vi "SET_PEG_LEG.vi"(10 "argv":string[](array[string]), 11 "args":u8) -> ()   [LabVIEW 2011]
uses:
  joe_johnson/peg_leg_state.ctl
panel:
  in  "StateMaps":cluster{"Name":string, "State":T1}[](array[cluster])=[{"Name"="up", "State"=enum."up"}, {"Name"="down", "State"=enum."down"}, {"Name"="unfold", "State"=enum."unfold"}]
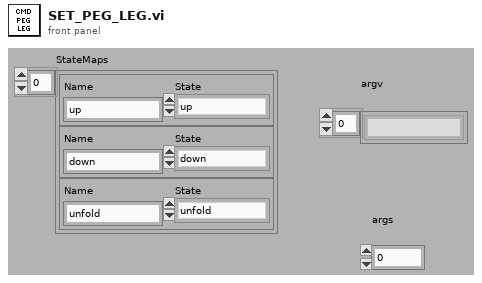
[diagram p1: front panel]
types:
  T1 = typedef "peg_leg_state.ctl" = enum16{"up", "down", "unfold", "manual"}
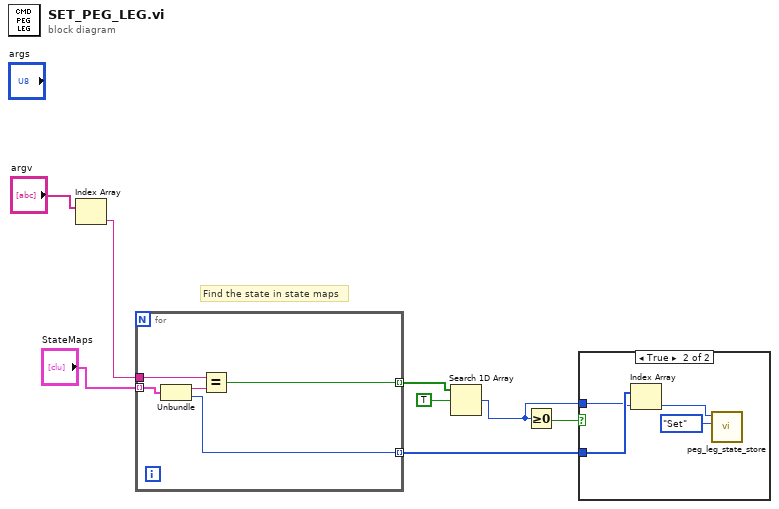
[diagram p0: block diagram]
diagram:
  # "Find the state in state maps"
  n1 = Index Array(array="argv") -> (element=w7:string)  [unwired: 1 in]
  n2 = for {
    tunnel: w7 -> [w13]
    tunnel: "StateMaps" -> [w12] mode=indexing
    tunnel: [w10] -> w5 mode=indexing
    tunnel: [w9] -> w2 mode=indexing
    n3 = Unbundle(w12) -> ("Name"=w11:string, "State"=w9:T1)
    n4 = Equal?(x=w13, y=w11) -> (x = y?=w10:bool)
  }
  n5 = Search 1D Array(1D array=w5, element=TRUE) -> (index of element=w1:i32)  [unwired: 1 out]
  n6 = Greater Or Equal To 0?(x=w1) -> (x >= 0?=w3:bool)
  n7 = case shown="True" w3 {
    tunnel: w2 -> [_ w17]
    tunnel: w1 -> [_ w16]
    frame False {
    }
    frame True {
      n8 = Index Array(array=w17, index=w16) -> (element=w15:T1)
      n9 = call "peg_leg_state_store.vi"("data_store_mode"=enum16{"Set", "Get"}."Set", "peg_leg_state"=w15) -> ()  [unwired: 8 in, 2 out]
    }
  }
